vi "Initialize.vi"(8 "error in (no error)":errorcluster, 9 "LTS state":T2, 10 "HTS state":T2, 11 "CurrentToField in":refnum<class "CurrentToField.lvclass">) -> (0 "error out":errorcluster, 1 "Ramp rate (T/min)":dbl, 2 "Setpoint (T)":dbl, 3 "CurrentToField out":refnum<class "CurrentToField.lvclass">, 5 "Ramp status":T1(ring))   [LabVIEW 2021, in "CurrentToField.lvclass"]
uses:
  CurrentToField.lvclass
  CurrentToField.lvclass/CurrentToField.ctl
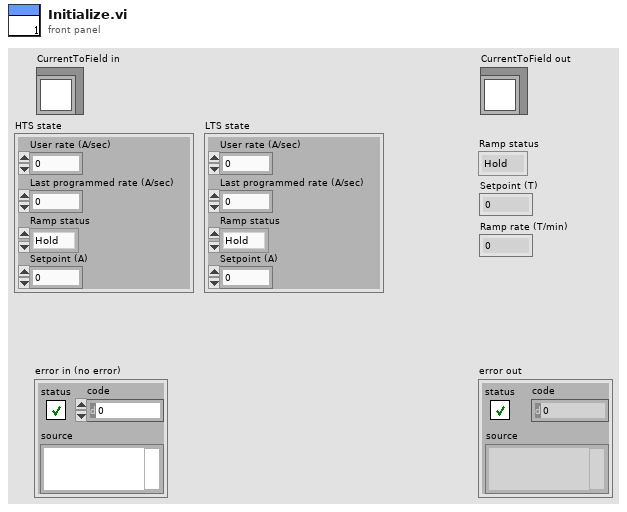
[diagram p1: front panel]
types:
  T1 = enum16{"Hold", "Ramp to zero", "Ramp to setpoint"}
  T2 = cluster{"User rate (A/sec)":dbl, "Last programmed rate (A/sec)":dbl, "Ramp status":enum16{"Hold", "Ramp to zero", "Ramp to setpoint"}, "Setpoint (A)":dbl}
  T3 = cluster{"HTS B_I0":dbl, "LTS B_I0":dbl, "HTS Bmax":dbl, "LTS Bmax":dbl, "Max combined rate (T/min)":dbl}
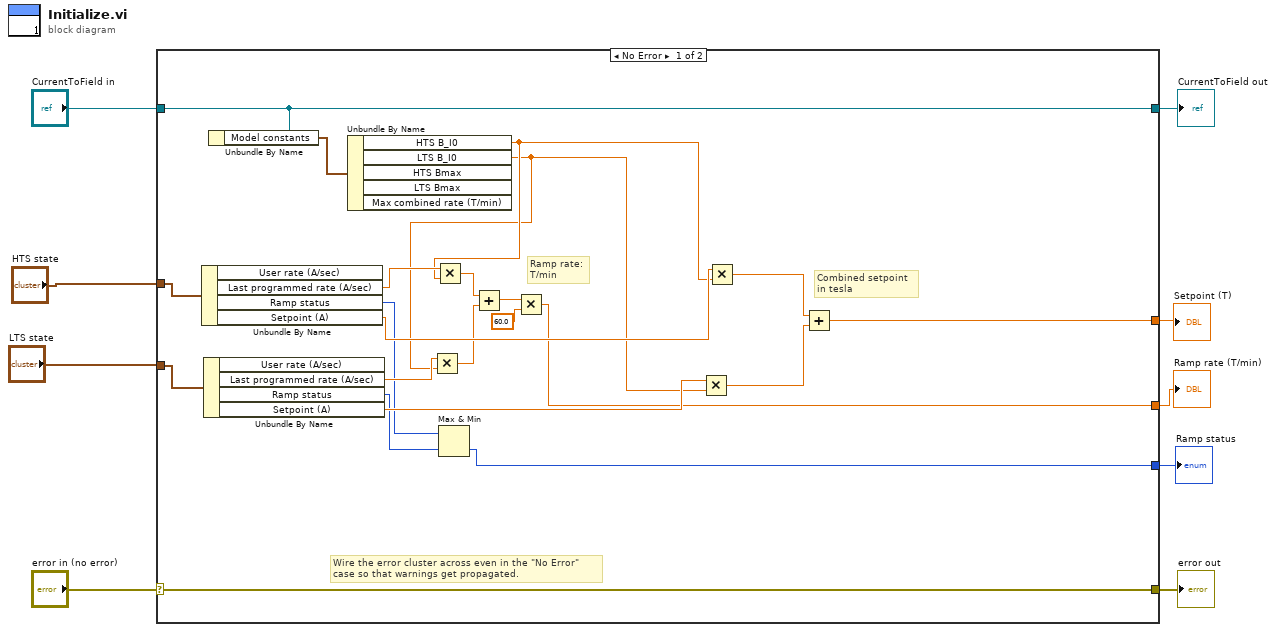
[diagram p0: block diagram]
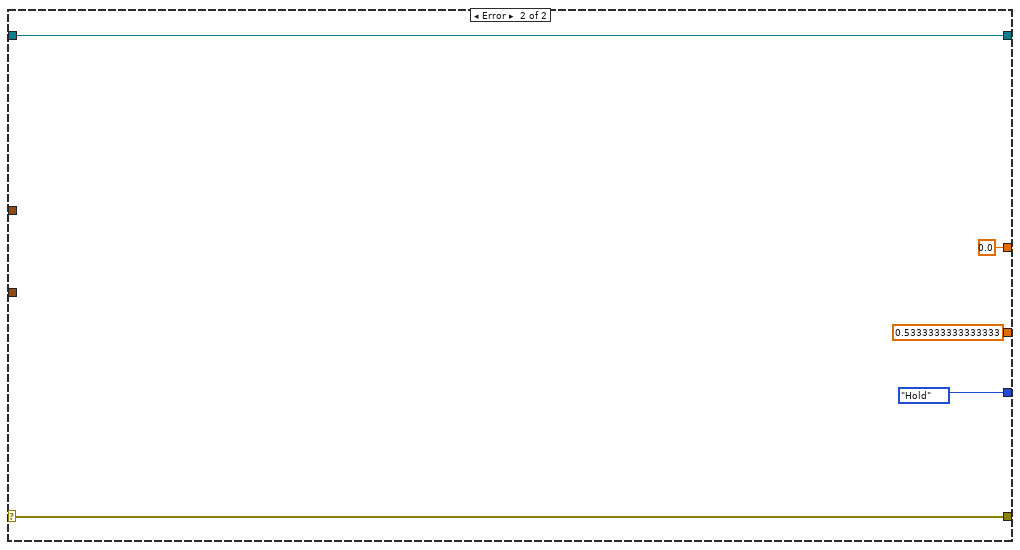
[diagram p2: hidden frame]
diagram:
  n1 = case shown="No Error" "error in (no error)" {
    selector: "error in (no error)" -> [w31 w36]
    tunnel: [w31 w36] -> w8
    tunnel: [w30 w35] -> w6
    tunnel: "CurrentToField in" -> [w30 w35]
    tunnel: "HTS state" -> [w28 _]
    tunnel: "LTS state" -> [w27 _]
    tunnel: [w12 T1."Hold" ("Ramp status")] -> w3
    tunnel: [w11 0.0] -> w2
    tunnel: [w10 0.5333333333333333] -> w1
    frame No Error {
      # "Ramp rate:\nT/min"
      # "Combined setpoint\nin tesla"
      # "Wire the error cluster across even in the \"No Error\"\ncase so that warnings get propagated."
      n2 = Unbundle By Name(w28) -> ("Last programmed rate (A/sec)"=w22:dbl, "Ramp status"=w14:T1, "Setpoint (A)"=w26:dbl)  [unwired: 1 out]
      n3 = Unbundle By Name(w27) -> ("Last programmed rate (A/sec)"=w21:dbl, "Ramp status"=w13:T1, "Setpoint (A)"=w25:dbl)  [unwired: 1 out]
      n4 = Unbundle By Name(w30) -> ("Model constants"=w29:T3)
      n5 = Unbundle By Name(w29) -> ("HTS B_I0"=w18:dbl, "LTS B_I0"=w17:dbl)  [unwired: 3 out]
      n6 = Multiply(x=w21, y=w17) -> (x*y=w19:dbl)
      n7 = Multiply(x=w22, y=w18) -> (x*y=w20:dbl)
      n8 = Max & Min(x=w14, y=w13) -> (min(x,y)=w12:u16)  [unwired: 1 out]
      n9 = Add(x=w20, y=w19) -> (x+y=w15:dbl)
      n10 = Multiply(x=w15, y=60.0) -> (x*y=w10:dbl)
      n11 = Multiply(x=w25, y=w17) -> (x*y=w24:dbl)
      n12 = Multiply(x=w26, y=w18) -> (x*y=w23:dbl)
      n13 = Add(x=w23, y=w24) -> (x+y=w11:dbl)
    }
    frame Error {
    }
  }
  "error out" <- w8
  "CurrentToField out" <- w6
  "Ramp status" <- w3
  "Setpoint (T)" <- w2
  "Ramp rate (T/min)" <- w1
